vi "User32.SendMessageA.vi"   [LabVIEW 2021]
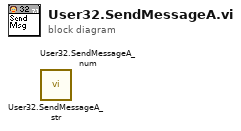
[diagram p0: block diagram]
diagram:
  n1 = call "User32.SendMessageA_str.vi"() -> ()  [unwired: 14 in, 2 out]
  n2 = call "User32.SendMessageA_num.vi"() -> ()  [unwired: 14 in, 2 out]
